vi "Autonomous Independent.vi"() -> ()   [LabVIEW 2018]
doc: "This VI is called when autonomous begins, and will automatically be terminated when autonomous ends. You can carry out timed or sensor driven robot movement independently without needing to return to the caller."
uses:
  Classes/StateMachine/StateMachine.lvclass
  Classes/Vision/Vision.lvclass
  Classes/Lift/Lift.lvclass
  <vilib>/Rock Robotics/WPI/Utilities/WPI_GetSetVariantRefNum.vi
  <vilib>/Rock Robotics/Network Tables/NT Read String.vi
  <vilib>/Rock Robotics/Network Tables/NT Write Numeric Array.vi
  <vilib>/Rock Robotics/WPI/RobotDrive/WPI_RobotDriveArcadeDrive_Standard(NoSaturation).vi
panel:
  out "Numeric":i32
  in  "stop":bool
  out "Current Movement, for debugging":T1 {"Y Joystick Value" scale=1.0..-1.0; "X Joystick Value" scale=-1.0..1.0}
  in  "Array of robot movements":T2(array[cluster])=[{"X Joystick Value"=0.39393939393939403, "Y Joystick Value"=0.0, "Delay (sec)"=1.0, "Movement Name"="turn"}, {"X Joystick Value"=-0.3737373737373737, "Y Joystick Value"=0.0, "Delay (sec)"=1.0, "Movement Name"="turn back"}] {"Y Joystick Value" scale=1.0..-1.0; "X Joystick Value" scale=-1.0..1.0}
  # "Be sure to right-click and choose Data Operations>>Make Current Value default if you want to save the array values with the VI"
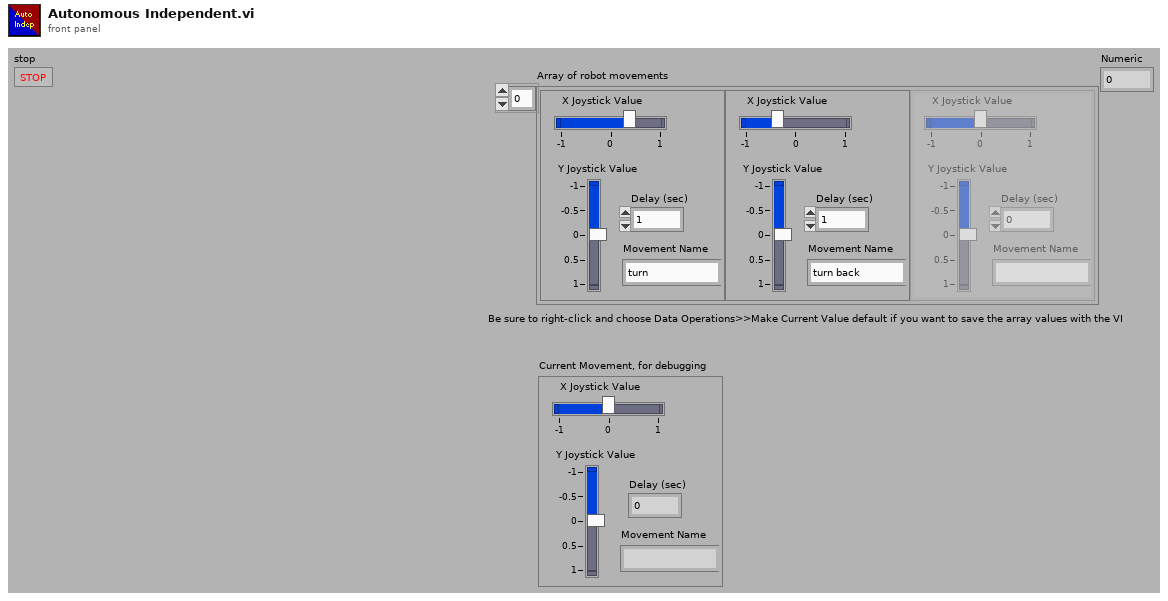
[diagram p1: front panel]
types:
  T1 = cluster{"X Joystick Value":dbl, "Y Joystick Value":dbl, "Delay (sec)":dbl, "Movement Name":string}
  T2 = cluster{"X Joystick Value":dbl, "Y Joystick Value":dbl, "Delay (sec)":dbl, "Movement Name":string}[]
  T3 = typedef "WPI_JoystickDevRef.ctl" = cluster{"Device":T4}
  T4 = typedef "WPI_JoystickDeviceEnum.ctl" = enum16{"USB 0", "USB 1", "USB 2", "USB 3", "USB 4", "USB 5"}
  T5 = cluster{"Button_Cargo_Load":bool, "Button_Rocket_1":bool, "Button_Rocket_2":bool, "Button_Rocket_3":bool}
  T6 = cluster{"Run Motionprofile?":bool, "Run Lift?":bool, "Run Vision?":bool, "Run Hatch Outtake?":bool, "Run Hatch Intake?":bool, "Which MotionProfile?":dbl, "Which LiftLevel?":dbl}
  T7 = typedef "WPI_RobotDriveDevRef.ctl" = cluster{"DevStatus":errorcluster, "Motors[]":T8[], "Square Inputs":bool, "Max Output":dbl}
  T8 = typedef "WPI_MotorControlDeviceRef.ctl" = cluster{"DeviceStatus":errorcluster, "Type":T9, "PWM":cluster{"PWM Channel":T10, "DeadBand":T11}, "CAN":cluster{"Device Number":u8, "SetOutput VI Ref":variant, "GetOutput VI Ref":variant, "Enable VI Ref":variant, "Disable VI Ref":variant, "Data":variant}, "Invert":bool, "DIO PWM":cluster{"PWM \"Enable\" Channel":T10, "DIOChannel":T12, "PWM Rate":dbl}}
  T9 = typedef "WPI_MotorControlType.ctl" = enum16{"PWM", "CAN", "DIO PWM"}
  T10 = typedef "FPGA_DIOPWMChannel.ctl" = enum8{"PWM 0", "PWM 1", "PWM 2", "PWM 3", "PWM 4", "PWM 5", "PWM 6", "PWM 7", "PWM 8", "PWM 9", "PWM MXP 0", "PWM MXP 1", "PWM MXP 2", "PWM MXP 3", "PWM MXP 4", "PWM MXP 5", "PWM MXP 6", "PWM MXP 7", "PWM MXP 8", "PWM MXP 9", "Invalid"}
  T11 = typedef "WPI_PWMDeadband.ctl" = cluster{"Name":string, "maxPositivePwm":i32, "minPositivePwm":i32, "centerPwm":i32, "maxNegativePwm":i32, "minNegativePwm":i32, "angularRange":u16}
  T12 = typedef "FPGA_DIOChannel.ctl" = enum8{"DIO 0", "DIO 1", "DIO 2", "DIO 3", "DIO 4", "DIO 5", "DIO 6", "DIO 7", "DIO 8", "DIO 9", "DIO MXP 0", "DIO MXP 1", "DIO MXP 2", "DIO MXP 3", "DIO MXP 4", "DIO MXP 5", "DIO MXP 6", "DIO MXP 7", "DIO MXP 8", "DIO MXP 9", "DIO MXP 10", "DIO MXP 11", "DIO MXP 12", "DIO MXP 13", "DIO MXP 14", "DIO MXP 15", "SPI Port CS1", "SPI Port CS2", "SPI Port CS3", "SPI Port MISO", "SPI Port MOSI", "Invalid"}
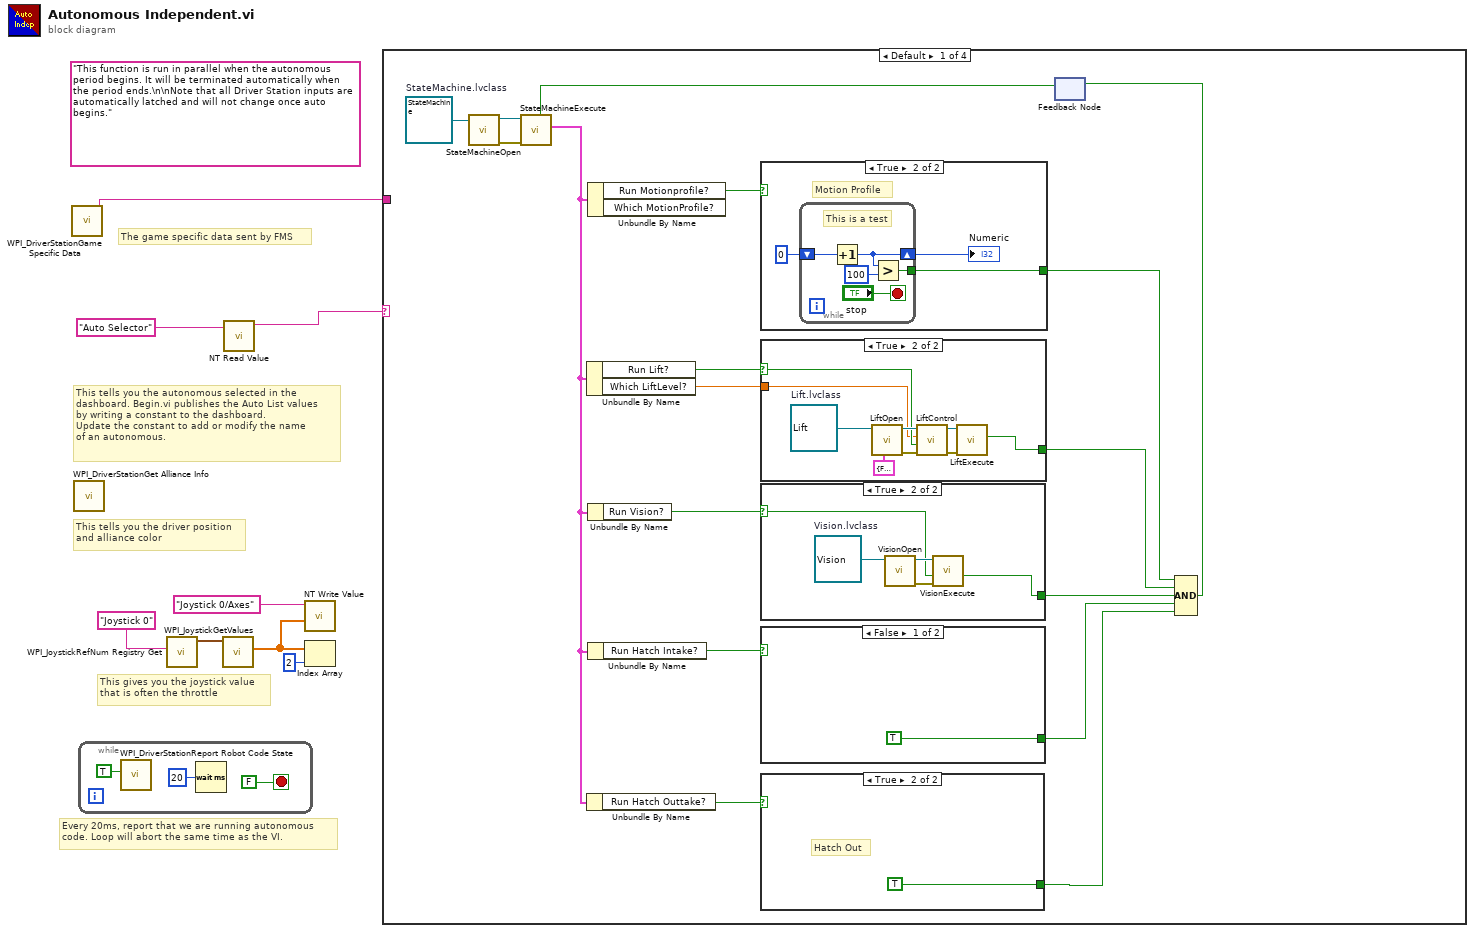
[diagram p0: block diagram]
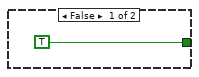
[diagram p2: hidden frame]
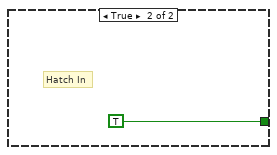
[diagram p3: hidden frame]
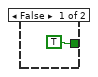
[diagram p4: hidden frame]
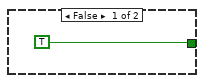
[diagram p5: hidden frame]
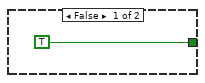
[diagram p6: hidden frame]
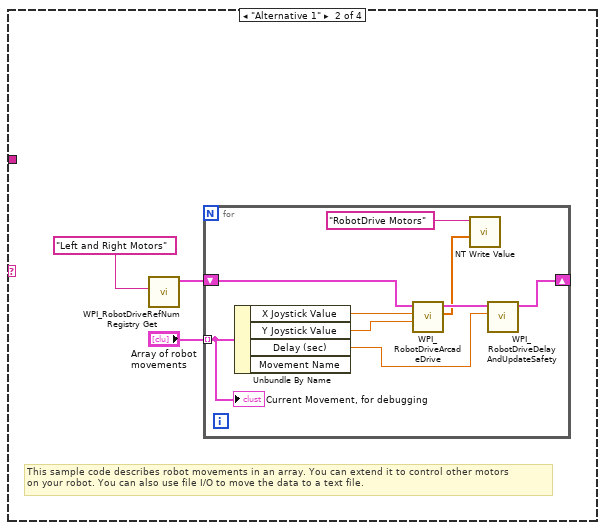
[diagram p7: hidden frame]
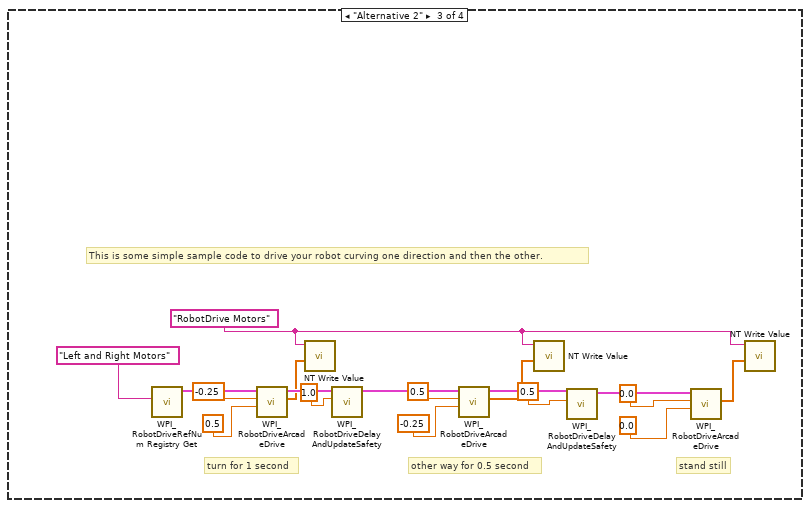
[diagram p8: hidden frame]
diagram:
  (unwired) "This function is run in parallel when the autonomous period begins. It will be terminated automatically when the period ends.\n\nNote that all Driver Station inputs are automatically latched and will not change once auto begins."
  # "The game specific data sent by FMS"
  # "This tells you the autonomous selected in the \ndashboard. Begin.vi publishes the Auto List values\nby writing a constant to the dashboard.\nUpdate the constant to add or modify the name\nof an autonomous."
  # "Every 20ms, report that we are running autonomous\ncode. Loop will abort the same time as the VI."
  # "This gives you the joystick value\nthat is often the throttle"
  # "This tells you the driver position\nand alliance color"
  n1 = call <vilib>:"WPI_DriverStationGame Specific Data.vi"() -> ("Game Specific Data"=w1:string)  [unwired: 11 in]
  n2 = call <vilib>:"WPI_DriverStationGet Alliance Info.vi"() -> ()  [unwired: 12 out]
  n3 = while {
    stop <- FALSE stop-if-true
    n4 = call <vilib>:"WPI_DriverStationReport Robot Code State.vi"("Autonomous"=TRUE) -> ()  [unwired: 10 in, 1 out]
    n5 = Wait (ms)(milliseconds to wait=u32 20) -> ()  [unwired: 1 out]
  }
  n6 = call <vilib>:"WPI_JoystickRefNum Registry Get.vi"("refnum name"="Joystick 0") -> ("JoystickDevRef"=w7:T3)  [unwired: 1 in, 9 out]
  n7 = call <vilib>:"WPI_JoystickGetValues.vi"("JoystickDevRef"=w7) -> ("Axes"=w3:dbl[])  [unwired: 6 in, 4 out]
  n8 = call-poly <vilib>:"NT Read Value.vi"("Name"="Auto Selector") -> ("String"=w4:string)  [unwired: 9 in, 1 out]
  n9 = call-poly <vilib>:"NT Write Value.vi"("Numeric Array"=w3, "Name"="Joystick 0/Axes") -> ()  [unwired: 9 in, 1 out]
  n10 = Index Array(array=w3, index=2) -> ()  [unwired: 1 out]
  n11 = case shown="Default" w4 {
    tunnel: w1 -> [_ _ _ _]
    frame Default {
      w22 = refnum<class "StateMachine.lvclass"> refnum  # StateMachine.lvclass
      n12 = call "StateMachineOpen.vi"("StateMachine in"=w22) -> ("error out"=w20:errorcluster, "StateMachine out"=w21:refnum<class "StateMachine.lvclass">)  [unwired: 9 in]
      n13 = feedback #1() -> (w13:bool)  [unwired: 1 in]
      n14 = call "StateMachineExecute.vi"("States finished?"=w13, "error in (no error)"=w20, "StateMachine in"=w21) -> ("output cluster"=w23:T6)  [unwired: 6 in, 2 out]
      n15 = Unbundle By Name(w23) -> ("Run Lift?"=w27:bool, "Which LiftLevel?"=w12:dbl)
      n16 = Unbundle By Name(w23) -> ("Run Hatch Outtake?"=w24:bool)
      n17 = Unbundle By Name(w23) -> ("Run Motionprofile?"=w28:bool)  [unwired: 1 out]
      n18 = Unbundle By Name(w23) -> ("Run Vision?"=w26:bool)
      n19 = Unbundle By Name(w23) -> ("Run Hatch Intake?"=w25:bool)
      n20 = case shown="True" w28 {
        tunnel: [TRUE w50] -> w19
        frame False {
        }
        frame True {
          # "Motion Profile"
          n21 = while {
            shift-right: [w55] -> w51
            shift-left: 0 -> [w56]
            tunnel: [w53] -> w50
            stop <- "stop" stop-if-true
            # "This is a test"
            n22 = Increment(x=w56) -> (x+1=w55:i32)
            n23 = Greater?(x=w55, y=100) -> (0:w53:bool)
          }
          "Numeric" <- w51
        }
      }
      n24 = case shown="True" w27 {
        selector: w27 -> [_ w44]
        tunnel: [TRUE w40] -> w18
        tunnel: w12 -> [_ w43]
        frame False {
        }
        frame True {
          w48 = refnum<class "Lift.lvclass"> refnum  # Lift.lvclass
          n25 = call "LiftOpen.vi"("Controller Values"=T5 {"Button_Cargo_Load"=FALSE, "Button_Rocket_1"=FALSE, "Button_Rocket_2"=FALSE, "Button_Rocket_3"=FALSE}, "Lift in"=w48) -> ("error out"=w46:errorcluster, "Lift out"=w45:refnum<class "Lift.lvclass">)  [unwired: 8 in]
          n26 = call "LiftControl.vi"("error in (no error)"=w46, "Autonomous?"=w44, "LiftLevel Auto?"=w43, "Lift in"=w45) -> ("error out"=w42:errorcluster, "Lift out"=w41:refnum<class "Lift.lvclass">)  [unwired: 6 in]
          n27 = call-dynamic "LiftExecute.vi"("error in (no error)"=w42, "Lift in"=w41) -> ("Setpoint reached?"=w40:bool)  [unwired: 7 in, 2 out]
        }
      }
      n28 = case shown="True" w26 {
        selector: w26 -> [_ w35]
        tunnel: [TRUE w34] -> w17
        frame False {
        }
        frame True {
          w38 = refnum<class "Vision.lvclass"> refnum  # Vision.lvclass
          n29 = call "VisionOpen.vi"("Vision in"=w38) -> ("error out"=w37:errorcluster, "Vision out"=w36:refnum<class "Vision.lvclass">)  [unwired: 9 in]
          n30 = call "VisionExecute.vi"("error in (no error)"=w37, "Vision enabled?"=w35, "Vision in"=w36) -> ("Vision Finished?"=w34:bool)  [unwired: 6 in, 2 out]
        }
      }
      n31 = case shown="False" w25 {
        tunnel: [TRUE TRUE] -> w16
        frame False {
        }
        frame True {
          # "Hatch In"
        }
      }
      n32 = case shown="True" w24 {
        tunnel: [TRUE TRUE] -> w15
        frame False {
        }
        frame True {
          # "Hatch Out"
        }
      }
      n33 = Compound Arithmetic op=AND(w19, w18, w17, w16, w15) -> (w14:bool)
      n34 = feedback-in #1(w14) -> ()
    }
    frame "Alternative 1" {
      # "This sample code describes robot movements in an array. You can extend it to control other motors\non your robot. You can also use file I/O to move the data to a text file."
      n35 = call <vilib>:"WPI_RobotDriveRefNum Registry Get.vi"("refnum name"="Left and Right Motors") -> ("RobotDriveDevRef"=w59:T7)  [unwired: 1 in, 9 out]
      n36 = for {
        shift-right: [w67] -> _
        shift-left: w59 -> [w68]
        tunnel: "Array of robot movements" -> [w63] mode=indexing
        n37 = Unbundle By Name(w63) -> ("X Joystick Value"=w66:dbl, "Y Joystick Value"=w65:dbl, "Delay (sec)"=w64:dbl)  [unwired: 1 out]
        n38 = call-poly <vilib>:"WPI_RobotDriveArcadeDrive.vi"("Y axis value"=w65, "X axis value"=w66, "RobotDriveDevRef"=w68) -> ("Motor Values"=w61:dbl[], "RobotDriveDevRef"=w69:T7)  [unwired: 1 in, 6 out]
        n39 = call-poly <vilib>:"NT Write Value.vi"("Numeric Array"=w61, "Name"="RobotDrive Motors") -> ()  [unwired: 9 in, 1 out]
        n40 = call <vilib>:"WPI_RobotDriveDelayAndUpdateSafety.vi"("Delay (s)"=w64, "RobotDriveDevRef"=w69) -> ("RobotDriveDevRef 2"=w67:T7)  [unwired: 8 in, 1 out]
        "Current Movement, for debugging" <- w63
      }
    }
    frame "Alternative 2" {
      w71 = "RobotDrive Motors" ("Name")
      # "This is some simple sample code to drive your robot curving one direction and then the other."
      # "stand still"
      # "other way for 0.5 second"
      # "turn for 1 second"
      n41 = call <vilib>:"WPI_RobotDriveRefNum Registry Get.vi"("refnum name"="Left and Right Motors") -> ("RobotDriveDevRef"=w87:T7)  [unwired: 1 in, 9 out]
      n42 = call-poly <vilib>:"WPI_RobotDriveArcadeDrive.vi"("Y axis value"=0.5 ("X axis value"), "X axis value"=-0.25, "RobotDriveDevRef"=w87) -> ("Motor Values"=w70:dbl[], "RobotDriveDevRef"=w80:T7)  [unwired: 1 in, 6 out]
      n43 = call-poly <vilib>:"NT Write Value.vi"("Numeric Array"=w70, "Name"=w71) -> ()  [unwired: 9 in, 1 out]
      n44 = call <vilib>:"WPI_RobotDriveDelayAndUpdateSafety.vi"("Delay (s)"=1.0, "RobotDriveDevRef"=w80) -> ("RobotDriveDevRef 2"=w81:T7)  [unwired: 8 in, 1 out]
      n45 = call-poly <vilib>:"WPI_RobotDriveArcadeDrive.vi"("Y axis value"=-0.25 ("X axis value"), "X axis value"=0.5, "RobotDriveDevRef"=w81) -> ("Motor Values"=w72:dbl[], "RobotDriveDevRef"=w82:T7)  [unwired: 1 in, 6 out]
      n46 = call-poly <vilib>:"NT Write Value.vi"("Numeric Array"=w72, "Name"=w71) -> ()  [unwired: 9 in, 1 out]
      n47 = call <vilib>:"WPI_RobotDriveDelayAndUpdateSafety.vi"("Delay (s)"=0.5, "RobotDriveDevRef"=w82) -> ("RobotDriveDevRef 2"=w83:T7)  [unwired: 8 in, 1 out]
      n48 = call-poly <vilib>:"WPI_RobotDriveArcadeDrive.vi"("Y axis value"=0.0 ("X axis value"), "X axis value"=0.0, "RobotDriveDevRef"=w83) -> ("Motor Values"=w73:dbl[])  [unwired: 1 in, 7 out]
      n49 = call-poly <vilib>:"NT Write Value.vi"("Numeric Array"=w73, "Name"=w71) -> ()  [unwired: 9 in, 1 out]
    }
    frame "Your Turn" {
    }
  }
